vi "Serialize.vi"(7 "MsgSerializer":refnum<class "MsgSerializer.XML.lvclass">, 8 "error in (no error)":errorcluster, 11 "Value":variant) -> (0 "error out":errorcluster, 3 "Serialized Message":string)   [LabVIEW 2020, in "Caraya.lvlib" / "MsgSerializer.XML.lvclass"]
uses:
  MsgSerializer.XML.lvclass
  C:/projects/caraya/src/classes/MsgSerializer/MsgSerializer.lvclass
  MsgSerializer.XML.lvclass/MsgSerializer.XML.ctl
  MsgSerializer/MsgSerializer.lvclass/MsgSerializer.ctl
  format -- enum.ctl
  <vilib>/Utility/VariantDataType/Type.ctl
  <vilib>/Utility/VariantDataType/VariantType.lvlib
  MsgSerializer/MsgSerializer.lvclass
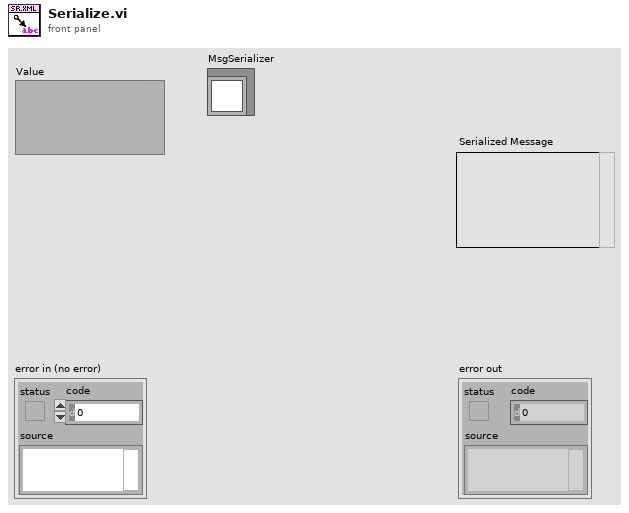
[diagram p1: front panel]
types:
  T1 = typedef "Caraya.lvlib/MsgSerializer.XML.lvclass/format -- enum.ctl" = enum16{"value", "tag", "property"}
  T2 = typedef "VariantType.lvlib/Type.ctl" = enum8{"Invalid Type", "Void", "I8", "I16", "I32", "I64", "U8", "U16", "U32", "U64", "Single Float", "Double Float", "Extended Float", "Single Complex", "Double Complex", "Extended Complex", "Enum U8", "Enum U16", "Enum U32", "Enum U64", "Single Float With Unit", "Double Float With Unit", "Extended Float With Unit", "Single Complex with Unit", "Double Complex with Unit", "Extended Complex with Unit", "Boolean", "String", "Path", "Picture", "Tag", "Array", "Cluster", "Variant", "LV Variant", "Waveform", "Timestamp", "Digital Waveform", "Digital Data", "ExpressData", "Refnum", "External Data", "VI", "Poly VI", "LabVIEW Class Instance", "Fixed Point"}
  T3 = typedef "TD_MDTFlavor.ctl" = enum16{"kUnknown", "OldDblWaveform", "I16Waveform", "DBLWaveform", "Unused(4)", "SGLWaveform", "Timestamp", "DigitalTable", "DigitalWaveform", "Dynamic Express", "ExtWaveform", "U8Waveform", "U16Waveform", "U32Waveform", "I8Waveform", "I32Waveform", "CSGWaveform", "CDBWaveform", "CXTWaveform", "I64Waveform", "U64Waveform"}
  T4 = typedef "VariantType.lvlib/RefnumType.ctl" = enum16{"NotARefnum", "UnknownRefnum", "Generic", "Datalog", "ByteStream", "Device", "Occurence", "TCPNetConnection", "Auto", "Menu", "Imaq", "Hardware", "DataSocket", "Visa", "IVI", "UDPNetConnection", "Notifier", "Queue", "Irda", "EventReg", "DotNet", "UserEvent", "Callback", "UNUSED_EMPTY_POSITION", "BlueToothNetConnection", "LVObjApp", "LVObjVI", "LVObjUnknown", "GenericClass", "UserDefinedRefnumTag", "DataValue", "RT FIFO", "TDMS File"}
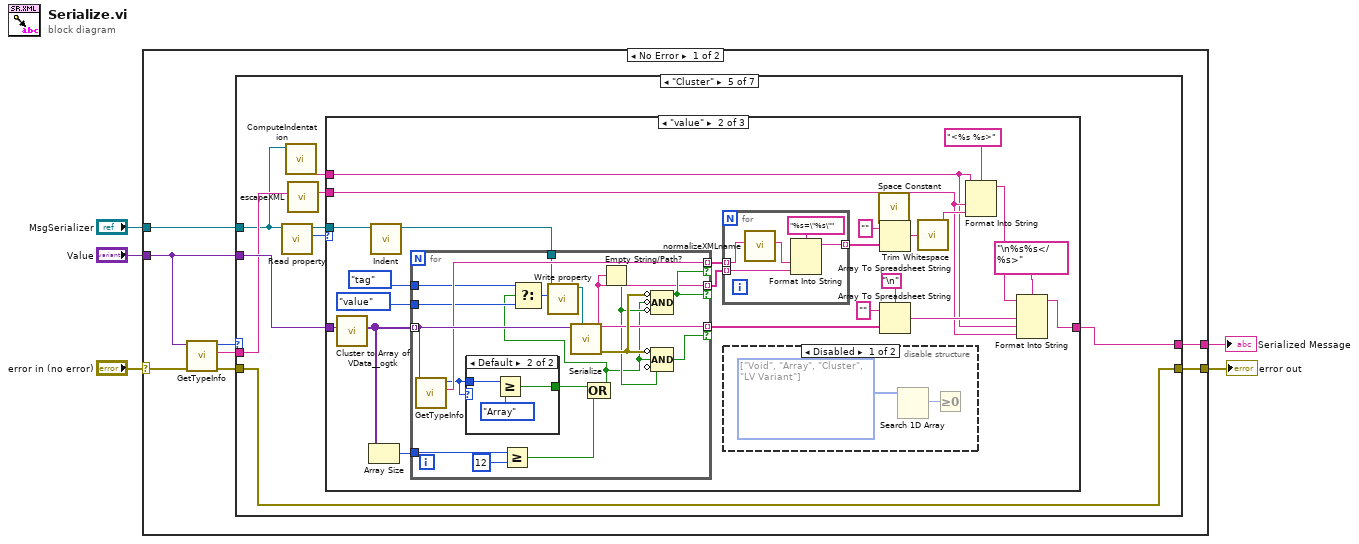
[diagram p0: block diagram]
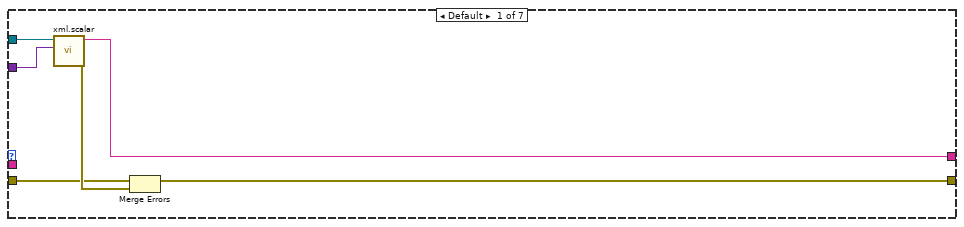
[diagram p2: hidden frame]
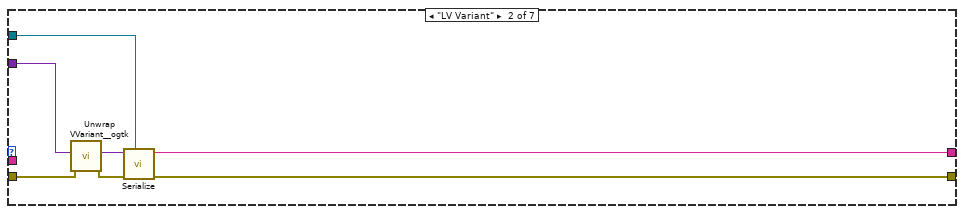
[diagram p3: hidden frame]
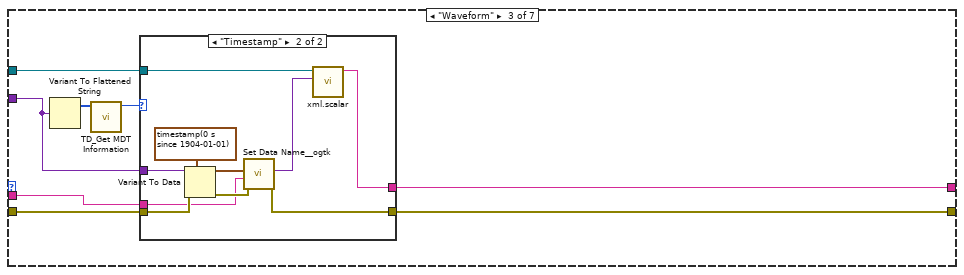
[diagram p4: hidden frame]
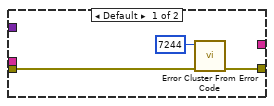
[diagram p5: hidden frame]
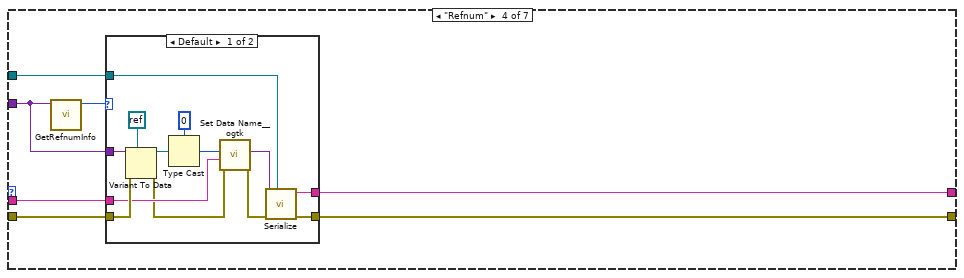
[diagram p6: hidden frame]
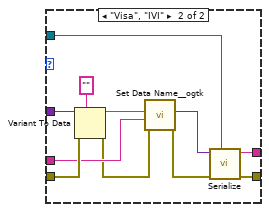
[diagram p7: hidden frame]
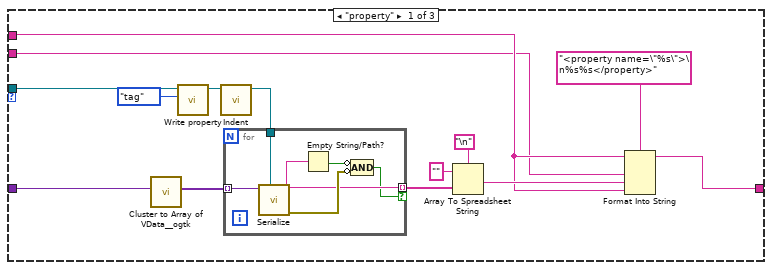
[diagram p8: hidden frame]
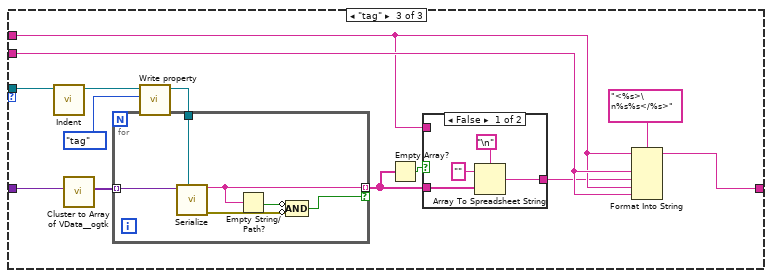
[diagram p11: hidden frame]
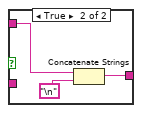
[diagram p12: hidden frame]
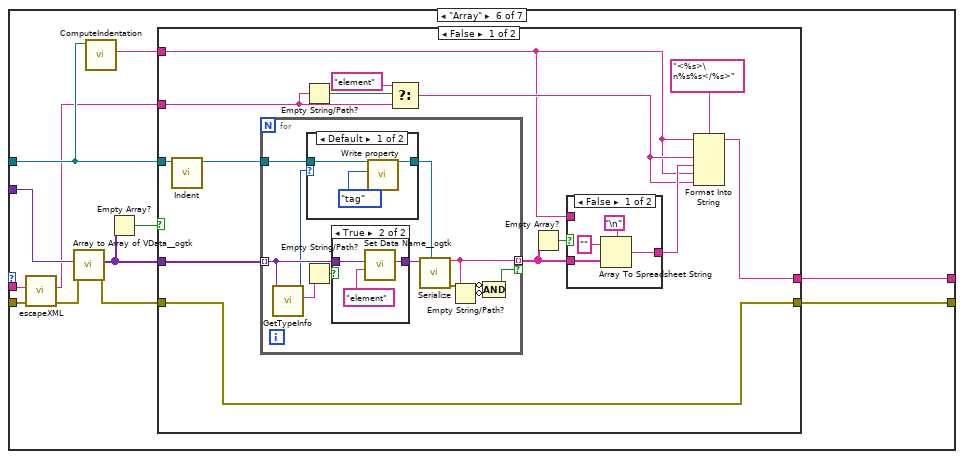
[diagram p13: hidden frame]
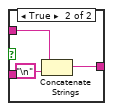
[diagram p14: hidden frame]
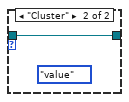
[diagram p15: hidden frame]
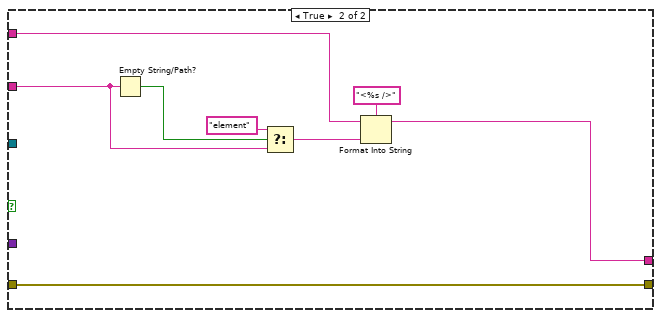
[diagram p17: hidden frame]
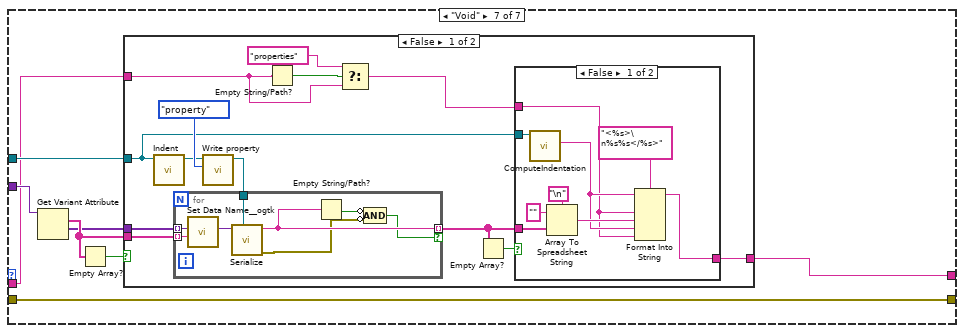
[diagram p18: hidden frame]
diagram:
  n1 = case shown="No Error" "error in (no error)" {
    selector: "error in (no error)" -> [w9 w283]
    tunnel: "MsgSerializer" -> [w7 _]
    tunnel: [w13 _] -> w4
    tunnel: "Value" -> [w12 _]
    tunnel: [w10 w283] -> w2
    frame No Error {
      n2 = call <vilib>:"GetTypeInfo.vi"("error in (no error)"=w9, "Variant"=w12) -> ("error out"=w8:errorcluster, "Name"=w6:string, "Type Enum"=w11:T2)  [unwired: 5 in, 2 out]
      n3 = case shown="\"Cluster\"" w11 {
        tunnel: [w17 w24 w30 w52 w84 w196 w247] -> w13
        tunnel: w12 -> [w18 w25 w28 w53 w87 w195 w252]
        tunnel: w7 -> [w19 w23 w29 w49 w80 w194 w246]
        tunnel: w8 -> [w15 w21 w32 w51 w86 w191 w248]
        tunnel: [w14 w20 w31 w50 w86 w186 w248] -> w10
        tunnel: w6 -> [_ _ w27 w48 w82 w192 w245]
        frame Default {
          n4 = call "xml.scalar.vi"("Value"=w18, "MsgSerializer.XML in"=w19) -> ("error out"=w16:errorcluster, "string"=w17:string)  [unwired: 8 in]
          n5 = Merge Errors(w15, w16) -> (w14:errorcluster)
        }
        frame "LV Variant" {
          n6 = call <userlib>:"Unwrap VVariant__ogtk.vi"("error in (no error)"=w21, "VVariant"=w25) -> ("error out"=w22:errorcluster, "Variant"=w26:variant)  [unwired: 8 in]
          n7 = call-dynamic "Serialize.vi"("MsgSerializer"=w23, "error in (no error)"=w22, "Value"=w26) -> ("error out"=w20:errorcluster, "Serialized Message"=w24:string)  [unwired: 7 in]
        }
        frame "Waveform" {
          n8 = Variant To Flattened String(Variant=w28) -> (1:w34:i16[])  [unwired: 1 out]
          n9 = call <vilib>:"TD_Get MDT Information.vi"("Type descriptor"=w34) -> ("MDT Flavor"=w33:T3)  [unwired: 9 in, 1 out]
          n10 = case shown="\"Timestamp\"" w33 {
            tunnel: w28 -> [_ w46]
            tunnel: [_ w38] -> w30
            tunnel: w32 -> [w36 w41]
            tunnel: [w37 w40] -> w31
            tunnel: w29 -> [_ w45]
            tunnel: w27 -> [_ w39]
            frame Default {
              n11 = call <vilib>:"Error Cluster From Error Code.vi"("error in (no error)"=w36, "error code (0)"=7244) -> ("error out"=w37:errorcluster)  [unwired: 7 in]
            }
            frame "Timestamp" {
              n12 = Variant To Data(error in=w41, type=timestamp(0 s since 1904-01-01) ("current time"), Variant=w46) -> (data=w44:timestamp, error out=w42:errorcluster)
              n13 = call <userlib>:"Set Data Name__ogtk.vi"("error in (no error)"=w42, "Data Name"=w39, "Data"=w44) -> ("error out"=w40:errorcluster, "Renamed Data"=w43:variant)  [unwired: 7 in]
              n14 = call "xml.scalar.vi"("Value"=w43, "MsgSerializer.XML in"=w45) -> ("string"=w38:string)  [unwired: 8 in, 1 out]
            }
          }
        }
        frame "Refnum" {
          n15 = call <vilib>:"GetRefnumInfo.vi"("Variant"=w53) -> ("ReferenceType"=w54:T4)  [unwired: 7 in, 3 out]
          n16 = case shown="Default" w54 {
            tunnel: w53 -> [w67 w77]
            tunnel: [w58 w71] -> w52
            tunnel: w51 -> [w66 w76]
            tunnel: [w57 w68] -> w50
            tunnel: w49 -> [w60 w72]
            tunnel: w48 -> [w61 w73]
            frame Default {
              n17 = Variant To Data(error in=w66, type=refnum<k0> refnum, Variant=w67) -> (data=w63:refnum<k0>, error out=w56:errorcluster)
              n18 = Type Cast(type=u32 0, x=w63) -> (*(type *) &x=w62:u32)
              n19 = call <userlib>:"Set Data Name__ogtk.vi"("error in (no error)"=w56, "Data Name"=w61, "Data"=w62) -> ("error out"=w55:errorcluster, "Renamed Data"=w59:variant)  [unwired: 7 in]
              n20 = call-dynamic "Serialize.vi"("MsgSerializer"=w60, "error in (no error)"=w55, "Value"=w59) -> ("error out"=w57:errorcluster, "Serialized Message"=w58:string)  [unwired: 7 in]
            }
            frame "Visa", "IVI" {
              n21 = Variant To Data(error in=w76, type="", Variant=w77) -> (data=w74:string, error out=w69:errorcluster)
              n22 = call <userlib>:"Set Data Name__ogtk.vi"("error in (no error)"=w69, "Data Name"=w73, "Data"=w74) -> ("error out"=w70:errorcluster, "Renamed Data"=w75:variant)  [unwired: 7 in]
              n23 = call-dynamic "Serialize.vi"("MsgSerializer"=w72, "error in (no error)"=w70, "Value"=w75) -> ("error out"=w68:errorcluster, "Serialized Message"=w71:string)  [unwired: 7 in]
            }
          }
        }
        frame "Cluster" {
          n24 = call "Read property.vi"("MsgSerializer.XMLProperty in"=w80) -> ("format"=w85:T1, "MsgSerializer.XMLProperty out"=w79:refnum<class "MsgSerializer.XML.lvclass">)  [unwired: 9 in]
          n25 = call "ComputeIndentation.vi"("MsgSerializer in"=w80) -> ("indentation"=w83:string)  [unwired: 10 in]
          n26 = call "escapeXML.vi"("Input String"=w82) -> ("XML-escaped String"=w81:string)  [unwired: 10 in]
          n27 = case shown="\"value\"" w85 {
            tunnel: w87 -> [w99 w131 w172]
            tunnel: w79 -> [w94 w129 w170]
            tunnel: w83 -> [w93 w108 w161]
            tunnel: w81 -> [w88 w109 w167]
            tunnel: [w96 w130 w171] -> w84
            frame "property" {
              n28 = call <userlib>:"Cluster to Array of VData__ogtk.vi"("Cluster"=w99) -> ("Array of VData"=w97:variant[])  [unwired: 9 in, 1 out]
              n29 = call "Write property.vi"("format"=format_--_enum."tag", "MsgSerializer.XMLProperty in"=w94) -> ("MsgSerializer.XMLProperty out"=w92:refnum<class "MsgSerializer.XML.lvclass">)  [unwired: 9 in]
              n30 = call "Indent.vi"("MsgSerializer in"=w92) -> ("MsgSerializer out"=w91:refnum<class "MsgSerializer.XML.lvclass">)  [unwired: 10 in]
              n31 = for {
                tunnel: w97 -> [w107] mode=indexing
                tunnel: [w103] -> w98 mode=indexing if=w102
                tunnel: w91 -> [w106]
                n32 = call-dynamic "Serialize.vi"("MsgSerializer"=w106, "Value"=w107) -> ("error out"=w104:errorcluster, "Serialized Message"=w103:string)  [unwired: 8 in]
                n33 = Empty String/Path?(string/path=w103) -> (empty?=w105:bool)
                n34 = Compound Arithmetic op=AND(invert w105, invert w104) -> (w102:bool)
              }
              n35 = Array To Spreadsheet String(delimiter (Tab)="\n", array=w98, 3:"" ("format string")) -> (spreadsheet string=w95:string)
              n36 = Format Into String(format string="<property name=\"%s\">\n%s%s</property>", initial string=w93, w88, w95, w93) -> (resulting string=w96:string)  [unwired: 1 in, 1 out]
            }
            frame "value" {
              n37 = call <userlib>:"Cluster to Array of VData__ogtk.vi"("Cluster"=w131) -> ("Array of VData"=w111:variant[])  [unwired: 9 in, 1 out]
              n38 = Array Size(array=w111) -> (size(s)=w110:i32)
              n39 = call "Indent.vi"("MsgSerializer in"=w129) -> ("MsgSerializer out"=w114:refnum<class "MsgSerializer.XML.lvclass">)  [unwired: 10 in]
              n40 = for {
                tunnel: w111 -> [w156] mode=indexing
                tunnel: [w142] -> w128 mode=indexing if=w152
                tunnel: [w142] -> w120 mode=indexing if=w154
                tunnel: [w155] -> w121 mode=indexing if=w154
                tunnel: w114 -> [w150]
                tunnel: format_--_enum."tag" ("format") -> [w149]
                tunnel: format_--_enum."value" ("format") -> [w148]
                tunnel: w110 -> [w146]
                n41 = call <vilib>:"GetTypeInfo.vi"("Variant"=w156) -> ("Name"=w155:string, "Type Enum"=w140:T2)  [unwired: 6 in, 3 out]
                n42 = case shown="Default" w140 {
                  tunnel: w140 -> [_ w159]
                  tunnel: [_ w157] -> w143
                  frame "Timestamp" {
                  }
                  frame Default {
                    n43 = Greater Or Equal?(x=w159, y=Type."Array") -> (x >= y?=w157:bool)
                  }
                }
                n44 = Greater Or Equal?(x=w146, y=12) -> (x >= y?=w144:bool)
                n45 = Compound Arithmetic op=OR(w143, w144) -> (w139:bool)
                n46 = Select(t=w149, s=w139, f=w148) -> (s? t:f=w147:T1)
                n47 = call "Write property.vi"("format"=w147, "MsgSerializer.XMLProperty in"=w150) -> ("MsgSerializer.XMLProperty out"=w151:refnum<class "MsgSerializer.XML.lvclass">)  [unwired: 9 in]
                n48 = call-dynamic "Serialize.vi"("MsgSerializer"=w151, "Value"=w156) -> ("error out"=w153:errorcluster, "Serialized Message"=w142:string)  [unwired: 8 in]
                n49 = Empty String/Path?(string/path=w142) -> (empty?=w141:bool)
                n50 = Compound Arithmetic op=AND(invert w153, invert w139, invert w141) -> (w154:bool)
                n51 = Compound Arithmetic op=AND(invert w153, w139, invert w141) -> (w152:bool)
              }
              n52 = for {
                tunnel: w121 -> [w135] mode=indexing
                tunnel: w120 -> [w138] mode=indexing
                tunnel: [w136] -> w116 mode=indexing
                n53 = call "normalizeXMLname.vi"("Input Attribute Name"=w135) -> ("Compliant Attribute Name"=w134:string)  [unwired: 10 in]
                n54 = Format Into String(format string="%s=\"%s\"", w134, w138) -> (resulting string=w136:string)  [unwired: 2 in, 1 out]
              }
              n55 = disable-structure shown="Disabled" {
                frame Disabled {
                  w133 = T2[] [enum."Void", enum."Array", enum."Cluster", enum."LV Variant"] items=["Invalid Type", "Void", "I8", "I16", "I32", "I64", "U8", "U16", "U32", "U64", "Single Float", "Double Float", "Extended Float", "Single Complex", "Double Complex", "Extended Complex", "Enum U8", "Enum U16", "Enum U32", "Enum U64", "Single Float With Unit", "Double Float With Unit", "Extended Float With Unit", "Single Complex with Unit", "Double Complex with Unit", "Extended Complex with Unit", "Boolean", "String", "Path", "Picture", "Tag", "Array", "Cluster", "Variant", "LV Variant", "Waveform", "Timestamp", "Digital Waveform", "Digital Data", "ExpressData", "Refnum", "External Data", "VI", "Poly VI", "LabVIEW Class Instance", "Fixed Point"]
                  n56 = Search 1D Array(1D array=w133) -> (index of element=w132:i32)  [unwired: 2 in]
                  n57 = Greater Or Equal To 0?(x=w132) -> ()  [unwired: 1 out]
                }
                frame Enabled {
                }
              }
              n58 = call <vilib>:"Space Constant.vi"() -> ("String"=w118:string)
              n59 = Array To Spreadsheet String(delimiter (Tab)=w118, array=w116, 3:"" ("format string")) -> (spreadsheet string=w119:string)
              n60 = Array To Spreadsheet String(delimiter (Tab)="\n", array=w128, 3:"" ("format string")) -> (spreadsheet string=w124:string)
              n61 = call <vilib>:"Trim Whitespace.vi"("string"=w119) -> ("trimmed string"=w115:string)  [unwired: 1 in]
              n62 = Format Into String(format string="<%s %s>", initial string=w108, w109, w115) -> (resulting string=w122:string)  [unwired: 1 in, 1 out]
              n63 = Format Into String(format string="\n%s%s</%s>", initial string=w122, w124, w108, w109) -> (resulting string=w130:string)  [unwired: 1 in, 1 out]
            }
            frame "tag" {
              n64 = call "Indent.vi"("MsgSerializer in"=w170) -> ("MsgSerializer out"=w166:refnum<class "MsgSerializer.XML.lvclass">)  [unwired: 10 in]
              n65 = call <userlib>:"Cluster to Array of VData__ogtk.vi"("Cluster"=w172) -> ("Array of VData"=w168:variant[])  [unwired: 9 in, 1 out]
              n66 = call "Write property.vi"("format"=format_--_enum."tag", "MsgSerializer.XMLProperty in"=w166) -> ("MsgSerializer.XMLProperty out"=w164:refnum<class "MsgSerializer.XML.lvclass">)  [unwired: 9 in]
              n67 = for {
                tunnel: w168 -> [w185] mode=indexing
                tunnel: [w180] -> w162 mode=indexing if=w183
                tunnel: w164 -> [w182]
                n68 = call-dynamic "Serialize.vi"("MsgSerializer"=w182, "Value"=w185) -> ("error out"=w184:errorcluster, "Serialized Message"=w180:string)  [unwired: 8 in]
                n69 = Empty String/Path?(string/path=w180) -> (empty?=w181:bool)
                n70 = Compound Arithmetic op=AND(invert w181, invert w184) -> (w183:bool)
              }
              n71 = Empty Array?(array=w162) -> (empty?=w163:bool)
              n72 = case shown="False" w163 {
                tunnel: [w174 w178] -> w160
                tunnel: w162 -> [w173 _]
                tunnel: w161 -> [_ w177]
                frame False {
                  n73 = Array To Spreadsheet String(delimiter (Tab)="\n", array=w173, 3:"" ("format string")) -> (spreadsheet string=w174:string)
                }
                frame True {
                  n74 = Concatenate Strings(w177, "\n" ("delimiter (Tab)")) -> (w178:string)
                }
              }
              n75 = Format Into String(format string="<%s>\n%s%s</%s>", initial string=w161, w167, w160, w161, w167) -> (resulting string=w171:string)  [unwired: 1 in, 1 out]
            }
          }
        }
        frame "Array" {
          n76 = call "escapeXML.vi"("Input String"=w192) -> ("XML-escaped String"=w190:string)  [unwired: 10 in]
          n77 = call <userlib>:"Array to Array of VData__ogtk.vi"("error in (no error)"=w191, "MultiD Array"=w195) -> ("error out"=w187:errorcluster, "1D Array of Variants"=w189:variant[])  [unwired: 8 in]
          n78 = call "ComputeIndentation.vi"("MsgSerializer in"=w194) -> ("indentation"=w193:string)  [unwired: 10 in]
          n79 = Empty Array?(array=w189) -> (empty?=w188:bool)
          n80 = case shown="False" w188 {
            tunnel: [w210 w244] -> w196
            tunnel: w194 -> [w202 _]
            tunnel: w193 -> [w197 w239]
            tunnel: w190 -> [w201 w238]
            tunnel: w189 -> [w200 _]
            tunnel: w187 -> [w199 w237]
            tunnel: [w199 w237] -> w186
            frame False {
              n81 = call "Indent.vi"("MsgSerializer in"=w202) -> ("MsgSerializer out"=w198:refnum<class "MsgSerializer.XML.lvclass">)  [unwired: 10 in]
              n82 = for {
                tunnel: w200 -> [w227] mode=indexing
                tunnel: [w221] -> w204 mode=indexing if=w222
                tunnel: w198 -> [w218]
                n83 = call <vilib>:"GetTypeInfo.vi"("Variant"=w227) -> ("Name"=w226:string, "Type Enum"=w220:T2)  [unwired: 6 in, 3 out]
                n84 = Empty String/Path?(string/path=w226) -> (empty?=w225:bool)
                n85 = case shown="Default" w220 {
                  tunnel: [w231 w232] -> w219
                  tunnel: w218 -> [w230 w232]
                  frame Default {
                    n86 = call "Write property.vi"("format"=format_--_enum."tag", "MsgSerializer.XMLProperty in"=w230) -> ("MsgSerializer.XMLProperty out"=w231:refnum<class "MsgSerializer.XML.lvclass">)  [unwired: 9 in]
                  }
                  frame "Cluster" {
                    (unwired) format_--_enum."value" ("format")
                  }
                }
                n87 = case shown="True" w225 {
                  tunnel: [w233 w236] -> w228
                  tunnel: w227 -> [w233 w235]
                  frame False {
                  }
                  frame True {
                    n88 = call <userlib>:"Set Data Name__ogtk.vi"("Data Name"="element" ("t"), "Data"=w235) -> ("Renamed Data"=w236:variant)  [unwired: 8 in, 1 out]
                  }
                }
                n89 = call-dynamic "Serialize.vi"("MsgSerializer"=w219, "Value"=w228) -> ("error out"=w224:errorcluster, "Serialized Message"=w221:string)  [unwired: 8 in]
                n90 = Empty String/Path?(string/path=w221) -> (empty?=w223:bool)
                n91 = Compound Arithmetic op=AND(invert w224, invert w223) -> (w222:bool)
              }
              n92 = Empty String/Path?(string/path=w201) -> (empty?=w207:bool)
              n93 = Select(t="element", s=w207, f=w201) -> (s? t:f=w205:string)
              n94 = Empty Array?(array=w204) -> (empty?=w203:bool)
              n95 = case shown="False" w203 {
                tunnel: [w212 w216] -> w208
                tunnel: w204 -> [w211 _]
                tunnel: w197 -> [_ w215]
                frame False {
                  n96 = Array To Spreadsheet String(delimiter (Tab)="\n", array=w211, 3:"" ("format string")) -> (spreadsheet string=w212:string)
                }
                frame True {
                  n97 = Concatenate Strings(w215, "\n" ("delimiter (Tab)")) -> (w216:string)
                }
              }
              n98 = Format Into String(format string="<%s>\n%s%s</%s>", initial string=w197, w205, w208, w197, w205) -> (resulting string=w210:string)  [unwired: 1 in, 1 out]
            }
            frame True {
              n99 = Empty String/Path?(string/path=w238) -> (empty?=w242:bool)
              n100 = Select(t="element", s=w242, f=w238) -> (s? t:f=w240:string)
              n101 = Format Into String(format string="<%s />", initial string=w239, w240) -> (resulting string=w244:string)  [unwired: 1 in, 1 out]
            }
          }
        }
        frame "Void" {
          n102 = Get Variant Attribute(Variant=w252) -> (names=w250:string[], values=w249:variant[])  [unwired: 3 in, 2 out]
          n103 = Empty Array?(array=w250) -> (empty?=w251:bool)
          n104 = case shown="False" w251 {
            tunnel: w250 -> [w264 _]
            tunnel: w249 -> [w265 _]
            tunnel: [w263 _] -> w247
            tunnel: w246 -> [w257 _]
            tunnel: w245 -> [w254 _]
            frame False {
              n105 = call "Indent.vi"("MsgSerializer in"=w257) -> ("MsgSerializer out"=w260:refnum<class "MsgSerializer.XML.lvclass">)  [unwired: 10 in]
              n106 = call "Write property.vi"("format"=format_--_enum."property", "MsgSerializer.XMLProperty in"=w260) -> ("MsgSerializer.XMLProperty out"=w261:refnum<class "MsgSerializer.XML.lvclass">)  [unwired: 9 in]
              n107 = for {
                tunnel: w261 -> [w279]
                tunnel: w265 -> [w282] mode=indexing
                tunnel: w264 -> [w280] mode=indexing
                tunnel: [w277] -> w259 mode=indexing if=w275
                n108 = call <userlib>:"Set Data Name__ogtk.vi"("Data Name"=w280, "Data"=w282) -> ("Renamed Data"=w281:variant)  [unwired: 8 in, 1 out]
                n109 = call-dynamic "Serialize.vi"("MsgSerializer"=w279, "Value"=w281) -> ("error out"=w276:errorcluster, "Serialized Message"=w277:string)  [unwired: 8 in]
                n110 = Empty String/Path?(string/path=w277) -> (empty?=w278:bool)
                n111 = Compound Arithmetic op=AND(invert w278, invert w276) -> (w275:bool)
              }
              n112 = Empty String/Path?(string/path=w254) -> (empty?=w256:bool)
              n113 = Select(t="properties" ("format string"), s=w256, f=w254) -> (s? t:f=w253:string)
              n114 = Empty Array?(array=w259) -> (empty?=w258:bool)
              n115 = case shown="False" w258 {
                tunnel: [w270 _] -> w263
                tunnel: w259 -> [w269 _]
                tunnel: w257 -> [w268 _]
                tunnel: w253 -> [w266 _]
                frame False {
                  n116 = call "ComputeIndentation.vi"("MsgSerializer in"=w268) -> ("indentation"=w267:string)  [unwired: 10 in]
                  n117 = Array To Spreadsheet String(delimiter (Tab)="\n", array=w269, 3:"" ("format string")) -> (spreadsheet string=w271:string)
                  n118 = Format Into String(format string="<%s>\n%s%s</%s>", initial string=w267, w266, w271, w267, w266) -> (resulting string=w270:string)  [unwired: 1 in, 1 out]
                }
                frame True {
                }
              }
            }
            frame True {
            }
          }
        }
      }
    }
    frame Error {
    }
  }
  "error out" <- w2
  "Serialized Message" <- w4
